vi "numCmd_ObtainQueue_Array.vi"(11 "Command Name":string) -> (0 "error out":errorcluster, 3 "queue out":refnum<queue>)   [LabVIEW 2019, in "Trajectory_Library.lvlib"]
uses:
  Trajectory_Library.lvlib
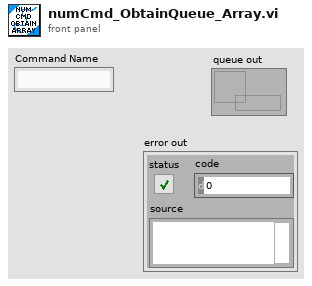
[diagram p1: front panel]
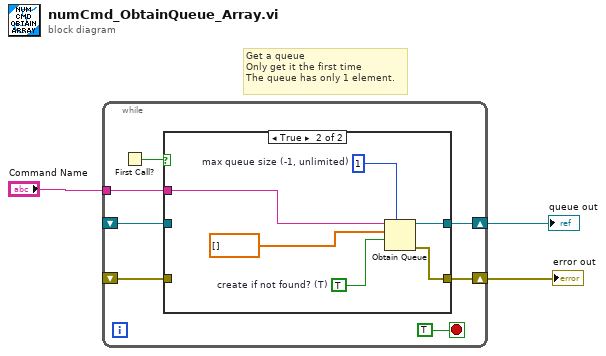
[diagram p0: block diagram]
diagram:
  # "Get a queue\nOnly get it the first time\nThe queue has only 1 element."
  n1 = while {
    tunnel: "Command Name" -> [w10]
    shift-right: [w5] -> w1
    shift-left: _ -> [w4]
    shift-right: [w7] -> w2
    shift-left: _ -> [w6]
    stop <- TRUE stop-if-true
    n2 = First Call?() -> (First Call?: T/F=w8:bool)
    n3 = case shown="True" w8 {
      tunnel: w10 -> [_ w16]
      tunnel: [w12 w15] -> w7
      tunnel: w6 -> [w12 _]
      tunnel: [w11 w14] -> w5
      tunnel: w4 -> [w11 _]
      frame False {
      }
      frame True {
        w17 = TRUE  # create if not found? (T)
        w18 = 1  # max queue size (-1, unlimited)
        n4 = Obtain Queue(max queue size (-1, unlimited)=w18, name (unnamed)=w16, element data type=dbl[] [], create if not found? (T)=w17) -> (queue out=w14:refnum<queue>, error out=w15:errorcluster)  [unwired: 1 in, 1 out]
      }
    }
  }
  "error out" <- w2
  "queue out" <- w1
